vi "RRTAlgorithm.vi"(0 "Dest x,y":dbl[](array[numeric]), 1 "Robot":T1={"id"=0, "function"=enum."Attacker", "x"=0.0, "y"=0.0, "orientation"=0.0, "v_tangent"=0.0, "v_normal"=0.0, "v_ang"=0.0, "kick_x"=0.0, "kick_z"=0.0, "dribble"=FALSE, "Timestamp"=timestamp(0 s since 1904-01-01), "estimatives"={"est_v_tangent"=0.0, "est_v_normal"=0.0, "est_vx"=0.0, "est_vy"=0.0, "Pos Robot Est"=[]}, "dest_x_kick"=0.0, "dest_y_kick"=0.0, "Gap Coord"=[], "States"=enum."Pass", "Path "=[], "Path  Smooth"=[], "Dest"=[], "vx_desired"=0.0, "vy_desired"=0.0, "slowBehavior"=FALSE, "VSSStates"=enum."Pass"}, 2 "WayPointProb":dbl, 3 "Path in \n(Smooth do Feedback Node)":dbl[][](array[numeric]), 4 "Step":dbl, 5 "GoalProb":dbl, 6 "Simple Path":dbl[][](array[numeric]), 7 "Ball":T7, 8 "Initial Pos x,y":dbl[](array[numeric]), 9 "our_robots":T1[](array[typedef]), 10 "Initial Pos 1,x,y,0":dbl[](array[numeric]), 11 "enemy_robots":T1[](array[typedef]), 12 "ignoreBall?":bool, 13 "Field Geomtery":u32[](array[numeric])) -> (16 "Path":dbl[][](array[numeric]))   [LabVIEW 2023]
uses:
  kD-tree/KD-Tree.ctl
  kD-tree/Node.ctl
  Vision_class/Old vision/SSL Detection Frame Simple Estimator Cameras VelCmd Folder/Core/AI Ball.ctl
  Vision_class/Old vision/Controls/AI Robot.ctl
  Vision_class/Old vision/Controls/Functions Enum.ctl
  Vision_class/Old vision/Controls/AttackerStates.ctl
  Vision_class/Old vision/Controls/PathDests.ctl
  Vision_class/Old vision/Controls/PathDest.ctl
  Navigation/VSSNavigation/VSSAttackerStates.ctl
  <vilib>/Analysis/_algsub.llb/Real Vector Norm.vi
  <vilib>/Analysis/NI_AALPro.lvlib
panel:
  out "Elapsed Time (s)":dbl
  out "New KD-Tree":T8
  out "x > y? 2":bool
  out "Modulo":dbl
  in  "threshold":dbl=80.0
  out "Time has Elapsed":bool
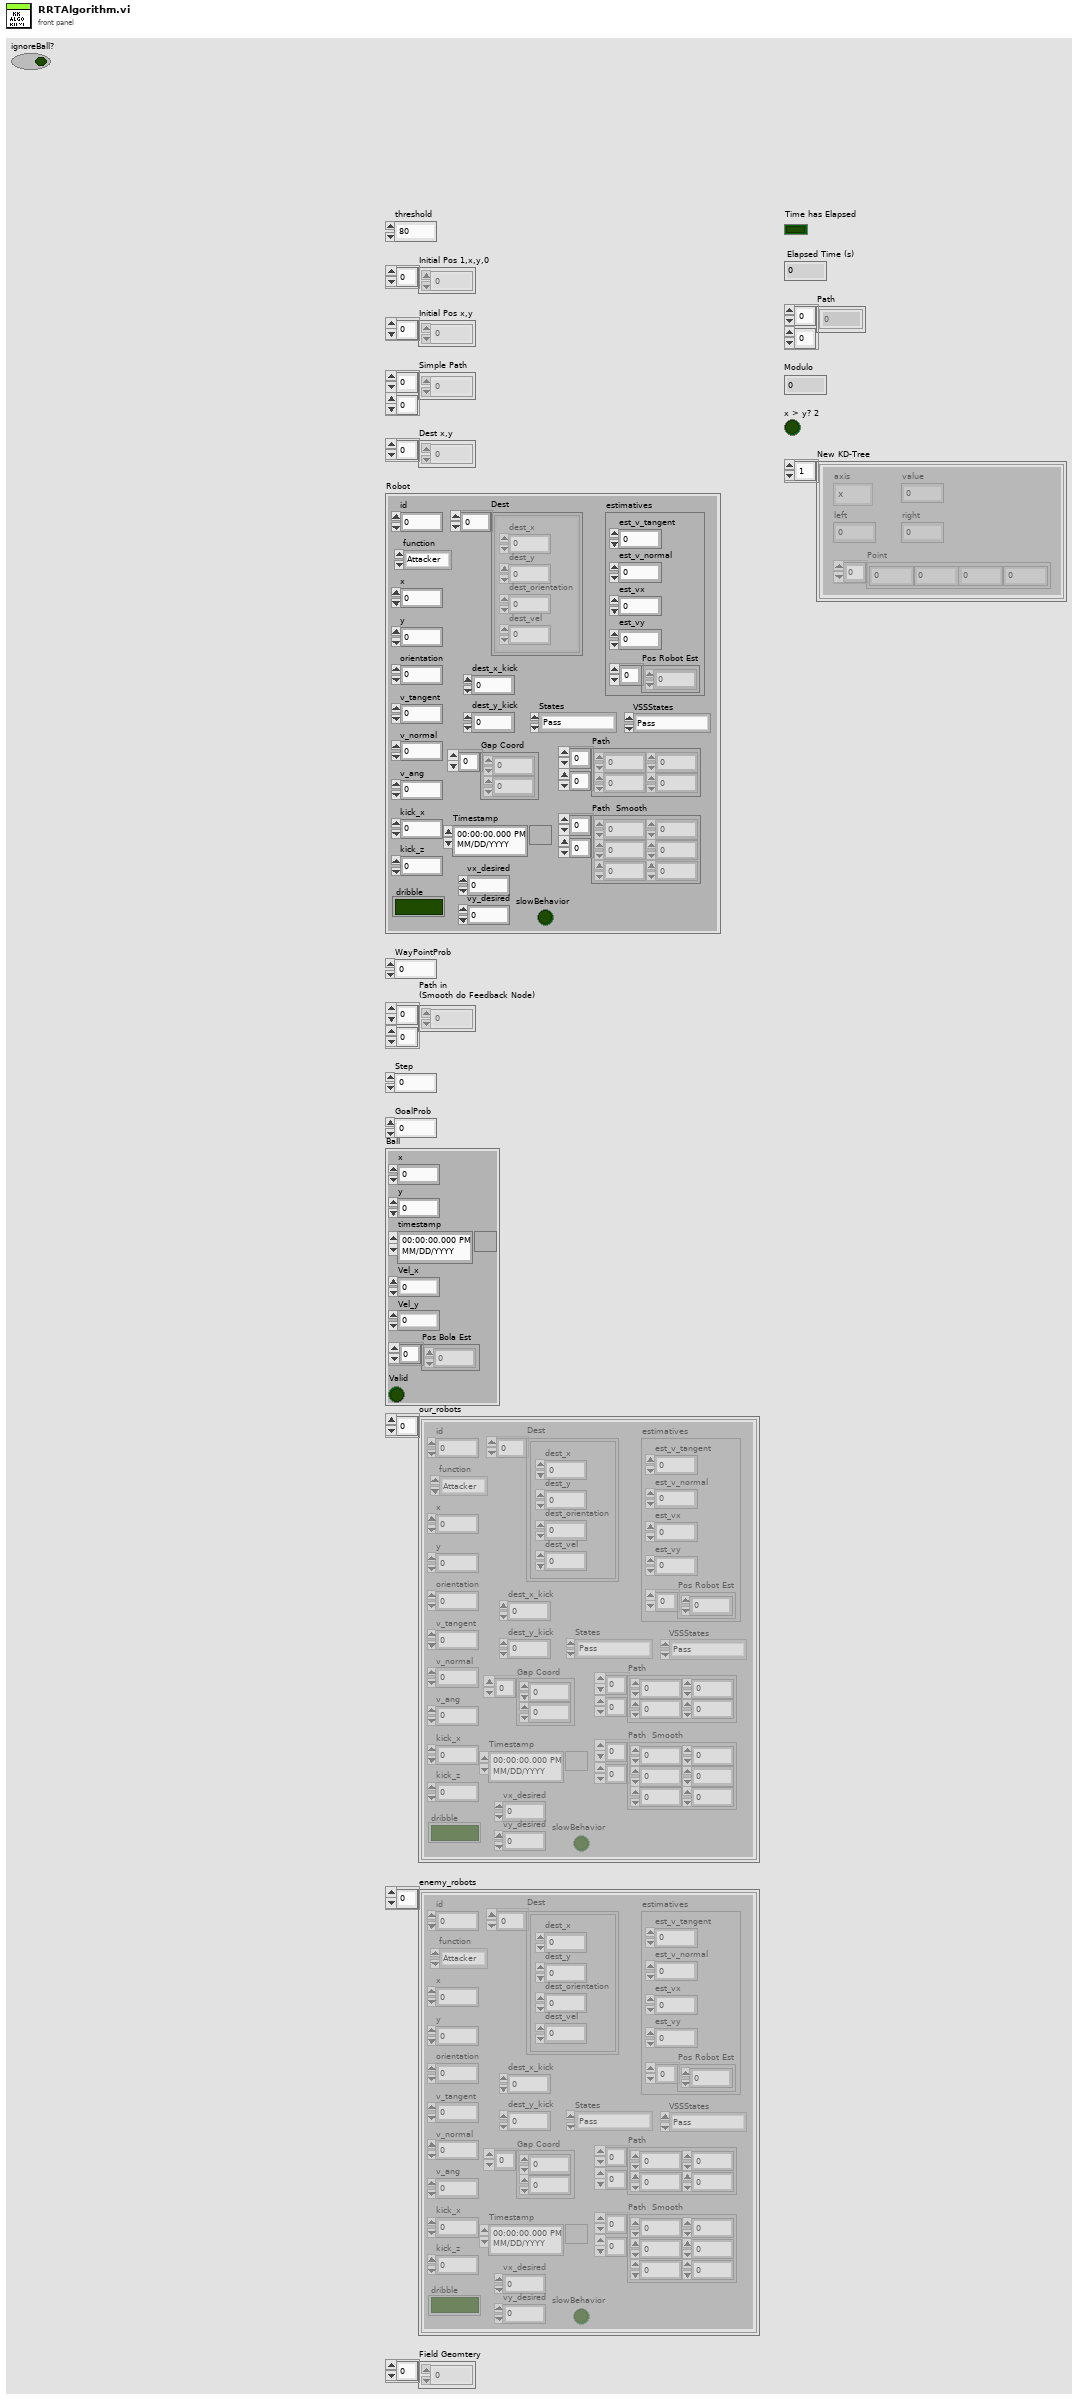
[diagram p1: front panel]
types:
  T1 = typedef "AI Robot.ctl" = cluster{"id":u32, "function":T2, "x":dbl, "y":dbl, "orientation":dbl, "v_tangent":dbl, "v_normal":dbl, "v_ang":dbl, "kick_x":dbl, "kick_z":dbl, "dribble":bool, "Timestamp":timestamp, "estimatives":cluster{"est_v_tangent":dbl, "est_v_normal":dbl, "est_vx":dbl, "est_vy":dbl, "Pos Robot Est":dbl[]}, "dest_x_kick":dbl, "dest_y_kick":dbl, "Gap Coord":dbl[], "States":T3, "Path ":dbl[][], "Path  Smooth":dbl[][], "Dest":T4, "vx_desired":dbl, "vy_desired":dbl, "slowBehavior":bool, "VSSStates":T6}
  T2 = typedef "Functions Enum.ctl" = enum16{"2nd Striker", "Attacker", "Goalie", "Defender", "Striker", "Goto 0", "Dummy", "Kicker", "ZigZag 0", "ZigZag 1", "ZigZag 2", "ZigZag 3", "ZigZag 4", "ZigZag 5", "ZigZag 6", "ZigZag 7", "ZigZag 8", ""}
  T3 = typedef "AttackerStates.ctl" = enum16{"Pass", "GoToTangent", "BallGetting", "GoToKick", ""}
  T4 = typedef "PathDests.ctl" = T5[]
  T5 = typedef "PathDest.ctl" = cluster{"dest_x":dbl, "dest_y":dbl, "dest_orientation":dbl, "dest_vel":dbl}
  T6 = typedef "VSSAttackerStates.ctl" = enum16{"Pass", "GoToTangent", "BallGetting", "GoToKick", "Rotate anti-clockwise", "Rotate Clockwise", ""}
  T7 = typedef "AI Ball.ctl" = cluster{"x":dbl, "y":dbl, "timestamp":timestamp, "Vel_x":dbl, "Vel_y":dbl, "Pos Bola Est":dbl[], "Valid":bool}
  T8 = typedef "KD-Tree.ctl" = T9[]
  T9 = typedef "Node.ctl" = cluster{"axis":enum16{"null", "x", "y"}, "value":dbl, "left":dbl, "right":dbl, "Point":dbl[]}
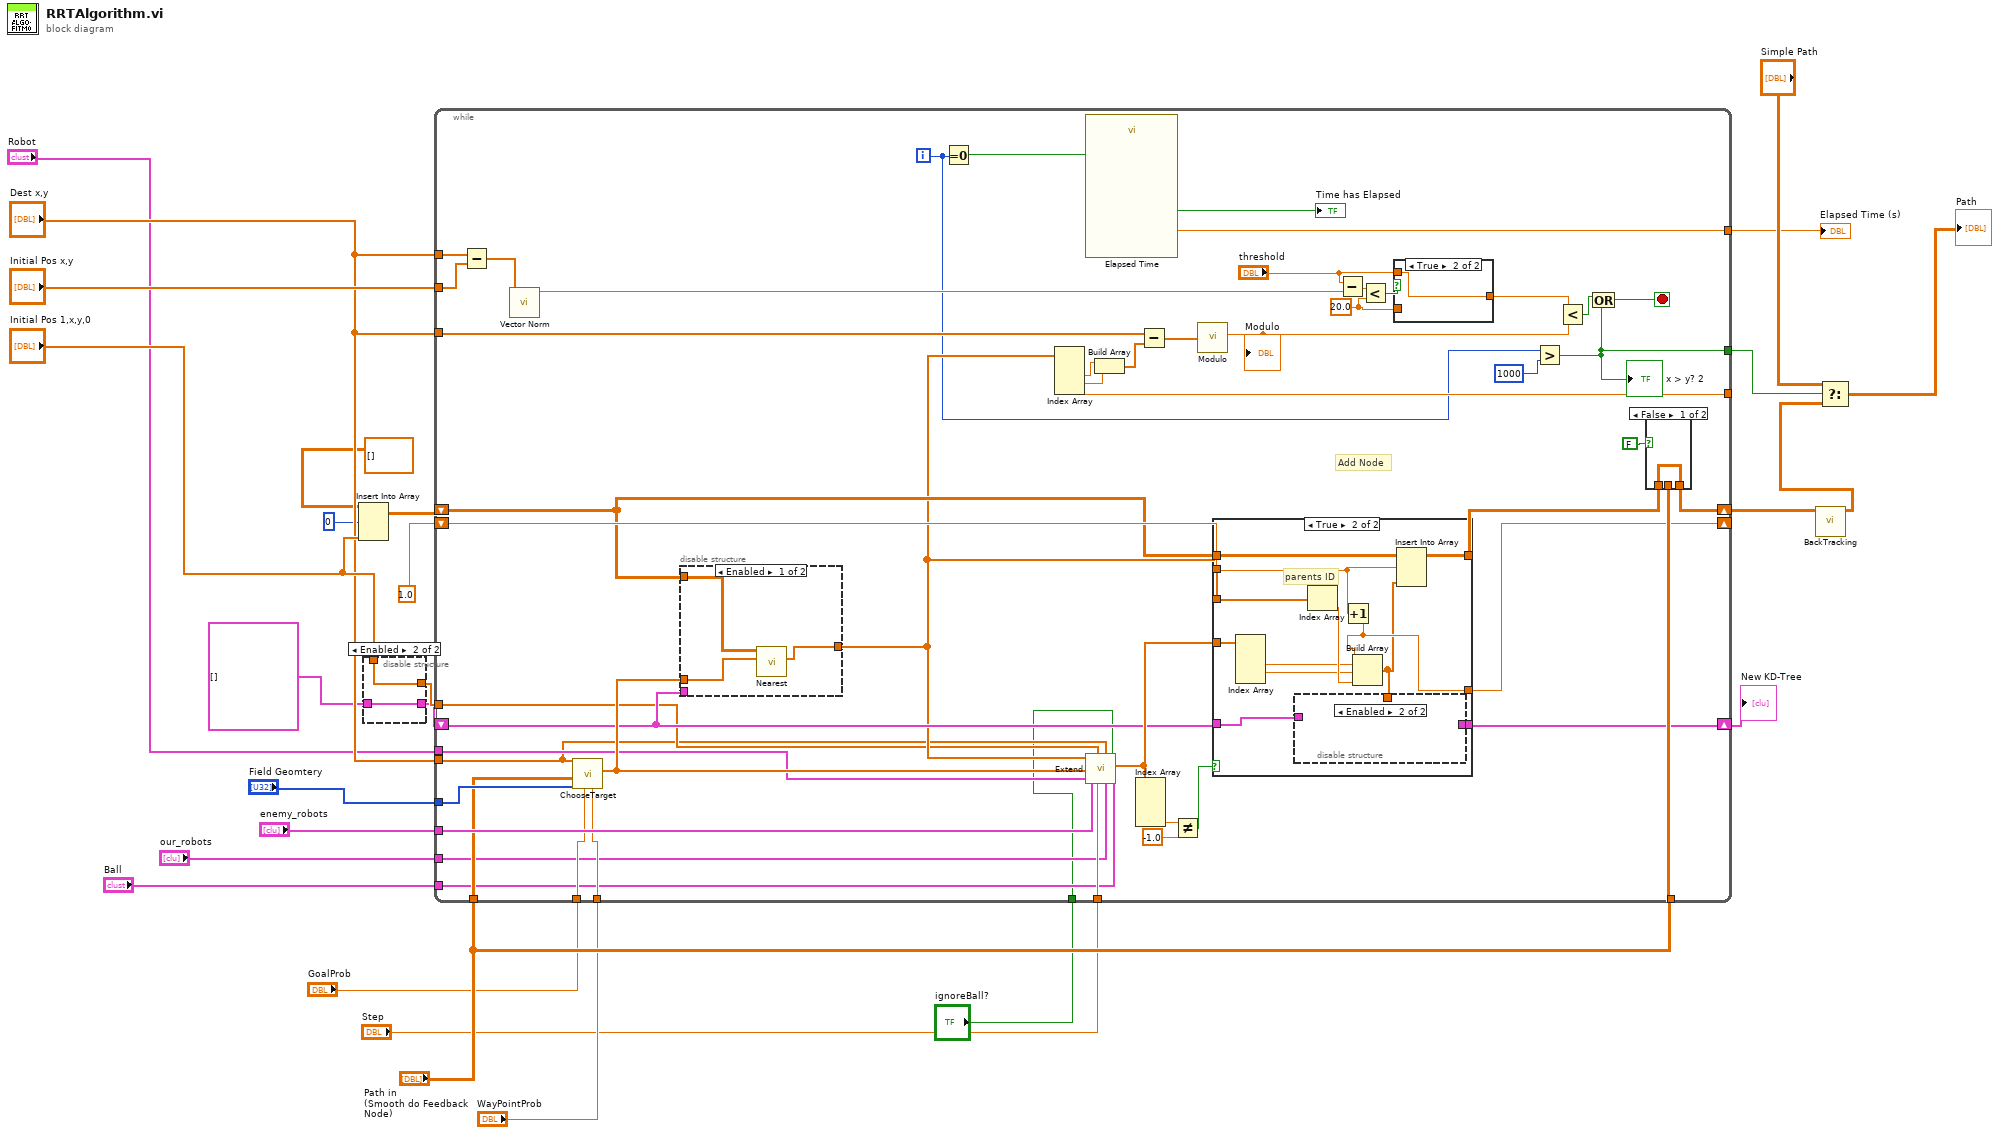
[diagram p0: block diagram]
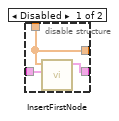
[diagram p2: hidden frame]
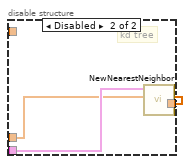
[diagram p3: hidden frame]
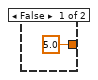
[diagram p4: hidden frame]
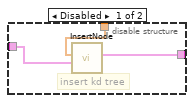
[diagram p7: hidden frame]
diagram:
  n1 = Insert Into Array(array=dbl[][] [] ("Pontos"), index (row)=0, new element="Initial Pos 1,x,y,0") -> (w4:dbl[][])  [unwired: 1 in]
  n2 = disable-structure shown="Enabled" {
    disable-tunnel: [w30 w32] -> w13
    disable-tunnel: T8 [] ("New KD-Tree") -> [w29 w32]
    disable-tunnel: "Initial Pos 1,x,y,0" -> [w28 w31]
    disable-tunnel: [w28 w31] -> w17
    frame Disabled {
      n3 = call "InsertFirstNode.vi"("New KD-Tree in"=w29, "Tree"=w28) -> ("New KD-Tree out"=w30:T8)  [unwired: 9 in]
    }
    frame Enabled {
    }
  }
  n4 = while {
    tunnel: "Dest x,y" -> [w82]
    tunnel: "Dest x,y" -> [w35]
    tunnel: "Field Geomtery" -> [w79]
    shift-right: [w63] -> w25
    shift-left: w4 -> [w62]
    tunnel: "enemy_robots" -> [w77]
    tunnel: "Step" -> [w76]
    shift-right: [w60] -> _
    shift-left: 1.0 -> [w67]
    tunnel: "Path in \n(Smooth do Feedback Node)" -> [w66]
    tunnel: "Path in \n(Smooth do Feedback Node)" -> [w65]
    tunnel: "GoalProb" -> [w58]
    tunnel: "WayPointProb" -> [w57]
    tunnel: [w55] -> _
    tunnel: "Dest x,y" -> [w54]
    shift-right: [w47] -> w12
    shift-left: w13 -> [w46]
    tunnel: [w44] -> w15
    tunnel: "Robot" -> [w42]
    tunnel: w17 -> [w41]
    tunnel: "Initial Pos x,y" -> [w40]
    tunnel: "our_robots" -> [w39]
    tunnel: "Ball" -> [w38]
    tunnel: [w34] -> w23
    tunnel: "ignoreBall?" -> [w33]
    i -> [w37]
    stop <- w71 stop-if-true
    w48 = 20.0 ("y")
    # "Add Node"
    n5 = Subtract(x=w54, y=w40) -> (x-y=w53:dbl[])
    n6 = call-poly <vilib>:"Vector Norm.vi"("Input Vector"=w53) -> ("norm"=w51:dbl)  [unwired: 9 in, 1 out]
    n7 = call "ChooseTarget.vi"("WayPointProb"=w57, "GoalProb"=w58, "Field Geometry"=w79, "WayPointCache"=w66, "Goal"=w35) -> ("Target"=w78:dbl[])  [unwired: 6 in]
    n8 = disable-structure shown="Enabled" {
      disable-tunnel: w78 -> [w86 w88]
      disable-tunnel: w62 -> [w85 _]
      disable-tunnel: w46 -> [_ w89]
      disable-tunnel: [w84 w87] -> w45
      frame Enabled {
        n9 = call "Nearest.vi"("Target"=w86, "Pontos"=w85) -> ("Nearest"=w84:dbl[])  [unwired: 9 in]
      }
      frame Disabled {
        # "kd tree"
        n10 = call "NewNearestNeighbor.vi"("q"=w88, "KD-Tree"=w89) -> ("Nearest"=w87:dbl[])  [unwired: 9 in]
      }
    }
    n11 = Equal To 0?(x=w37) -> (x = 0?=w43:bool)
    n12 = Index Array(array=w45) -> (element #2=w70:dbl, element #3=w69:dbl, element #4=w55:dbl)  [unwired: 4 in, 1 out]
    n13 = call "Elapsed Time"("Auto Reset"=w43) -> ("Elapsed Time (s)"=w44:dbl, "Time has Elapsed"=→"Time has Elapsed":bool)  [unwired: 11 in, 6 out]
    n14 = call "Extend.vi"("Ball"=w38, "ignoreBall?"=w33, "our_robots"=w39, "Goal"=w35, "Step"=w76, "Initial State"=w41, "enemy_robots"=w77, "Robot in"=w42, "Target"=w78, "Nearest"=w45) -> ("New State"=w72:dbl[])  [unwired: 1 in]
    n15 = Build Array(w70, w69) -> (w68:dbl[])
    n16 = Index Array(array=w72) -> (element #4=w75:dbl)  [unwired: 4 in, 3 out]
    n17 = Subtract(x=w82, y=w68) -> (x-y=w83:dbl[])
    n18 = Not Equal?(x=w75, y=-1.0) -> (x != y?=w73:bool)
    n19 = call "Modulo.vi"("2D vector"=w83) -> ("Modulo"=w81:dbl)  [unwired: 10 in]
    "Modulo" <- w81
    n20 = case shown="True" w73 {
      tunnel: w62 -> [w96 w108]
      tunnel: [w96 w104] -> w64
      tunnel: w72 -> [_ w107]
      tunnel: w67 -> [w95 w103]
      tunnel: w45 -> [_ w106]
      tunnel: [w95 w98] -> w60
      tunnel: [w94 w102] -> w47
      tunnel: w46 -> [w94 w101]
      frame False {
      }
      frame True {
        # "parents ID"
        n21 = Index Array(array=w107) -> (element #2=w100:dbl, element #3=w99:dbl)  [unwired: 4 in, 2 out]
        n22 = Index Array(array=w106) -> (element=w105:dbl)  [unwired: 1 in]
        n23 = Increment(x=w103) -> (x+1=w98:dbl)
        n24 = Build Array(w98, w100, w99, w105) -> (w97:dbl[])
        n25 = disable-structure shown="Enabled" {
          disable-tunnel: [w111 _] -> w102
          disable-tunnel: w101 -> [w110 _]
          disable-tunnel: w97 -> [w109 _]
          frame Disabled {
            # "insert kd tree"
            n26 = call "InsertNode.vi"("KD-Tree"=w110, "New Node"=w109) -> ("New KD-Tree"=w111:T8)  [unwired: 9 in]
          }
          frame Enabled {
          }
        }
        n27 = Insert Into Array(array=w108, index (row)=w103, new element=w97) -> (w104:dbl[][])  [unwired: 1 in]
      }
    }
    n28 = Subtract(x="threshold", y=w51) -> (x-y=w49:dbl)
    n29 = Less?(x=w49, y=w48) -> (x < y?=w50:bool)
    n30 = case shown="True" w50 {
      tunnel: [5.0 ("threshold") w91] -> w80
      tunnel: "threshold" -> [_ w91]
      tunnel: w48 -> [_ _]
      frame False {
      }
      frame True {
      }
    }
    n31 = Greater?(x=w37, y=1000) -> (0:w34:bool)
    "x > y? 2" <- w34
    n32 = Less?(x=w81, y=w80) -> (x < y?=w56:bool)
    n33 = Compound Arithmetic op=OR(w56, w34) -> (w71:bool)
    n34 = case shown="False" FALSE {
      tunnel: w65 -> [_ w93]
      tunnel: [w92 w93] -> w63
      tunnel: w64 -> [w92 _]
      frame False {
      }
      frame True {
      }
    }
  }
  "New KD-Tree" <- w12
  "Elapsed Time (s)" <- w15
  n35 = call "BackTracking.vi"("Pontos"=w25) -> ("Path"=w27:dbl[][])  [unwired: 9 in, 1 out]
  n36 = Select(t="Simple Path", s=w23, f=w27) -> (s? t:f=→"Path":dbl[][])
